vi "Read relayQueue.vi"(8 "error in (no error)":errorcluster, 11 "RelayAppender in":refnum<class "RelayAppender.lvclass">) -> (0 "error out":errorcluster, 2 "relayQueue":refnum<queue>, 3 "RelayAppender out":refnum<class "RelayAppender.lvclass">)   [LabVIEW 2026, in "Lumberjack.lvlib" / "RelayAppender.lvclass"]
doc: "Return the owned relay queue (queue mode) so the application can dequeue Statements. In message mode the returned refnum is invalid (message-mode relays deliver via the consumer enqueuer instead) (SRS-LMBR-025)."
uses:
  RelayAppender.lvclass
  TypeDefs/Statement.ctl
  TypeDefs/Severity.ctl
  RelayAppender.lvclass/RelayAppender.ctl
  Lumberjack.lvlib
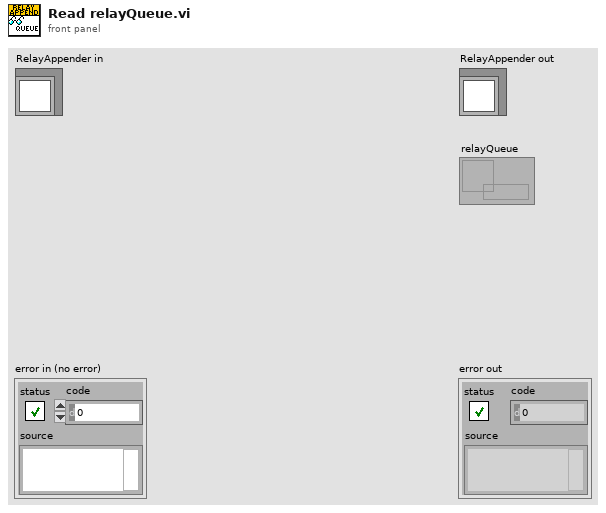
[diagram p1: front panel]
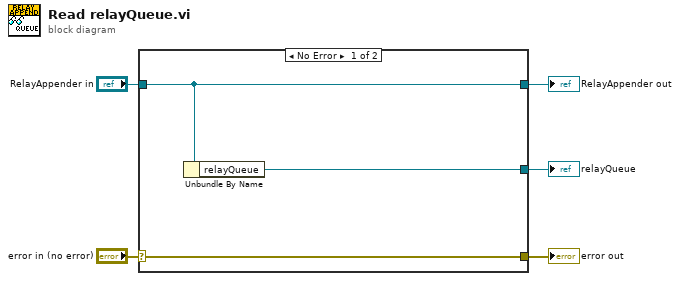
[diagram p0: block diagram]
diagram:
  n1 = case shown="No Error" "error in (no error)" {
    selector: "error in (no error)" -> [w8 w9]
    tunnel: [w8 w9] -> w4
    tunnel: [w7 w10] -> w2
    tunnel: "RelayAppender in" -> [w7 w10]
    tunnel: [w6 _] -> w1
    frame No Error {
      n2 = Unbundle By Name(w7) -> ("relayQueue"=w6:refnum<queue>)
    }
    frame Error {
    }
  }
  "error out" <- w4
  "RelayAppender out" <- w2
  "relayQueue" <- w1
